vi "StartMainGUI.vi"(8 "ErrorIn":errorcluster, 9 "MsTimeout(-1)":i32=-1, 11 "ReferenceIn":refnum<class "TemplateGUI.lvclass">) -> (0 "ErrorOut":errorcluster, 2 "TimedOut":bool, 3 "ReferenceOut":refnum<class "TemplateGUI.lvclass">, 5 "EventFromProcess":refnum<user-event>)   [LabVIEW 2021, in "TemplateGUI.lvlib" / "TemplateGUI.lvclass"]
doc: "Looks up an existing object matching object name or creates a new object and returns a refnum you can use when calling other class methods.\n\nObjects created with this VI should be destroyed using this class Delete VI."
uses:
  TemplateGUI.lvclass
  TemplateGUI.lvclass/TemplateGUI.ctl
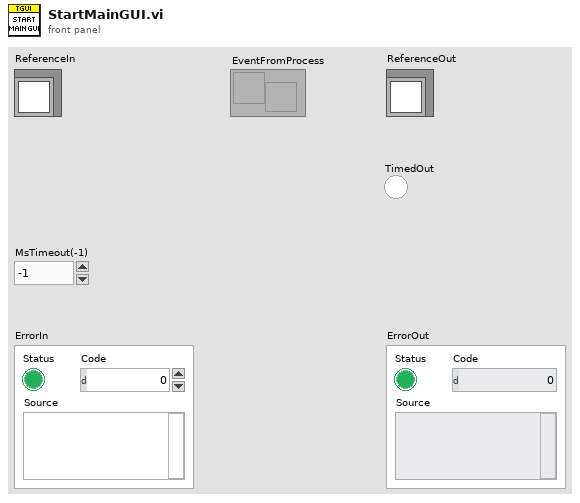
[diagram p1: front panel]
types:
  T1 = enum16{"ReadRepository", "CreateNew", "CreateOrLookUpExisting", "ReadRepositoryAndDestroy"}
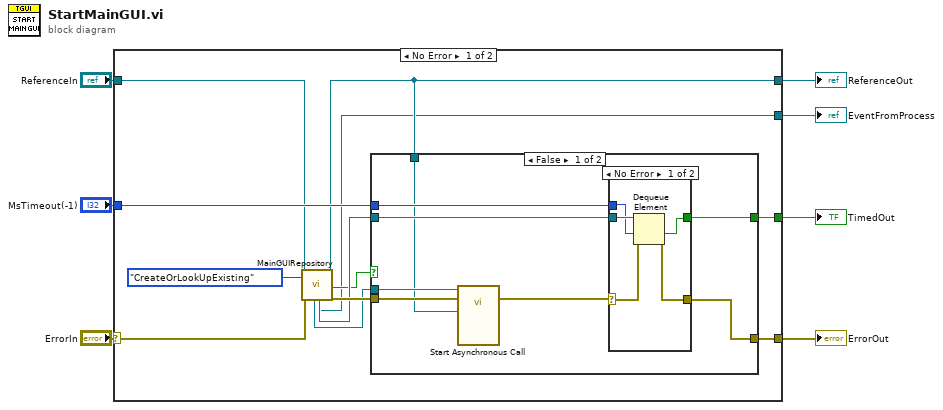
[diagram p0: block diagram]
diagram:
  n1 = case shown="No Error" "ErrorIn" {
    selector: "ErrorIn" -> [w18 w36]
    tunnel: [w19 w36] -> w6
    tunnel: [w12 w35] -> w4
    tunnel: "ReferenceIn" -> [w10 w35]
    tunnel: "MsTimeout(-1)" -> [w16 _]
    tunnel: [w15 _] -> w2
    tunnel: [w9 _] -> w1
    frame No Error {
      n2 = call "MainGUIRepository.vi"("reference in"=w10, "Action(ReadRepository)"=T1."CreateOrLookUpExisting", "Error In"=w18) -> ("ProcessViRef"=w14:refnum<vi>, "EventFromProcess"=w9:refnum<user-event>, "ProcessSyncQueue"=w13:refnum<queue>, "reference out"=w12:refnum<class "TemplateGUI.lvclass">, "ProcessAlreadyStarted"=w11:bool, "Error Out"=w17:errorcluster)  [unwired: 9 in, 2 out]
      n3 = case shown="False" w11 {
        tunnel: w16 -> [w24 _]
        tunnel: [w23 _] -> w15
        tunnel: [w27 w34] -> w19
        tunnel: w17 -> [w26 w34]
        tunnel: w14 -> [w21 _]
        tunnel: w13 -> [w22 _]
        tunnel: w12 -> [w20 _]
        frame False {
          n4 = call-by-ref "Start Asynchronous Call"(reference=w21, error in=w26, "reference in"=w20) -> (error out=w25:errorcluster)  [unwired: 17 in, 3 out]
          n5 = case shown="No Error" w25 {
            tunnel: w22 -> [w30 _]
            tunnel: w24 -> [w28 _]
            tunnel: [w29 _] -> w23
            selector: w25 -> [w32 w33]
            tunnel: [w31 w33] -> w27
            frame No Error {
              n6 = Dequeue Element(queue=w30, timeout in ms (-1)=w28, error in (no error)=w32) -> (timed out?=w29:bool, error out=w31:errorcluster)  [unwired: 2 out]
            }
            frame Error {
            }
          }
        }
        frame True {
          # "Process Already started.\nThis option will only be used togeather with the\naction: \"CreateOrLookUpExisting\""
        }
      }
    }
    frame Error {
    }
  }
  "ErrorOut" <- w6
  "ReferenceOut" <- w4
  "TimedOut" <- w2
  "EventFromProcess" <- w1
